vi "GPSPathTracker.vi"() -> ()   [LabVIEW 2024]
uses:
  <vilib>/Instr/_visa.llb/VISA Configure Serial Port (Instr).vi
  <vilib>/Utility/file.llb/Read Delimited Spreadsheet (DBL).vi
panel:
  in  "Steer Selector":enum32{"Stanley Method", "Pure Pursuit"}(radio)
  in  "Ld(m)":dbl=2.5 format="%#_13g"
  out "GPS":T1(graph)
  out "Tracking_Err(m)":dbl
  out "GPS_Steer_CMD(Deg)":dbl
  in  "Input_Spd(kph)":dbl
  out "RDDF_Velocity":dbl
  out "Output_Spd_CMD(%)":dbl
  out "Path_lat_arr":dbl[](array[numeric])
  out "Path_long_arr":dbl[](array[numeric])
  out "Path_Vel_arr":dbl[](array[numeric])
  out "WP_no.":i32
  out "Path_Evt_arr":dbl[](array[numeric])
  out "Evt":dbl
  in  "Map Refresh":bool
  out "X_lat_path_Full":dbl[](array[numeric])
  out "vel. path":dbl[](array[numeric])
  out "Y_long_path_Full":dbl[](array[numeric])
  out "Evt.Arr":dbl[](array[numeric])
  in  "COM7":refnum<visa-resource-name>="COM3" caption="GPS_Com."
  out "GPS_Speed(kph)":dbl format="%#_g kph"
  out "UTM Y(N) INS":dbl format="%#_13g"
  out "UTM X(E) INS":dbl format="%#_13g"
  out "True_Heading(deg)":dbl format="%#_15g"
  out "Latitude(deg)":dbl
  out "Logitude(deg)":dbl
  out "Altitude(m)":dbl
  in  "Stop":bool
  in  "RDDF":path=path "C:/Users/JungiHong/OneDrive/Hongik/HI-RACE/2026-01/ExperimentModules/GPSPathTracking/230305.txt"
  in  "k(Gain)":dbl=1.0 format="%#_13g"
  out "yi1":dbl=4158092.273483
  out "xi1":dbl=316694.021153
  out "yi":dbl=4158092.273483
  out "xi":dbl=316694.021153
  out "NMEA_Raw_Data":string
  out "CTE":dbl=20.227725199184242
  # "GPS 연결 포트"
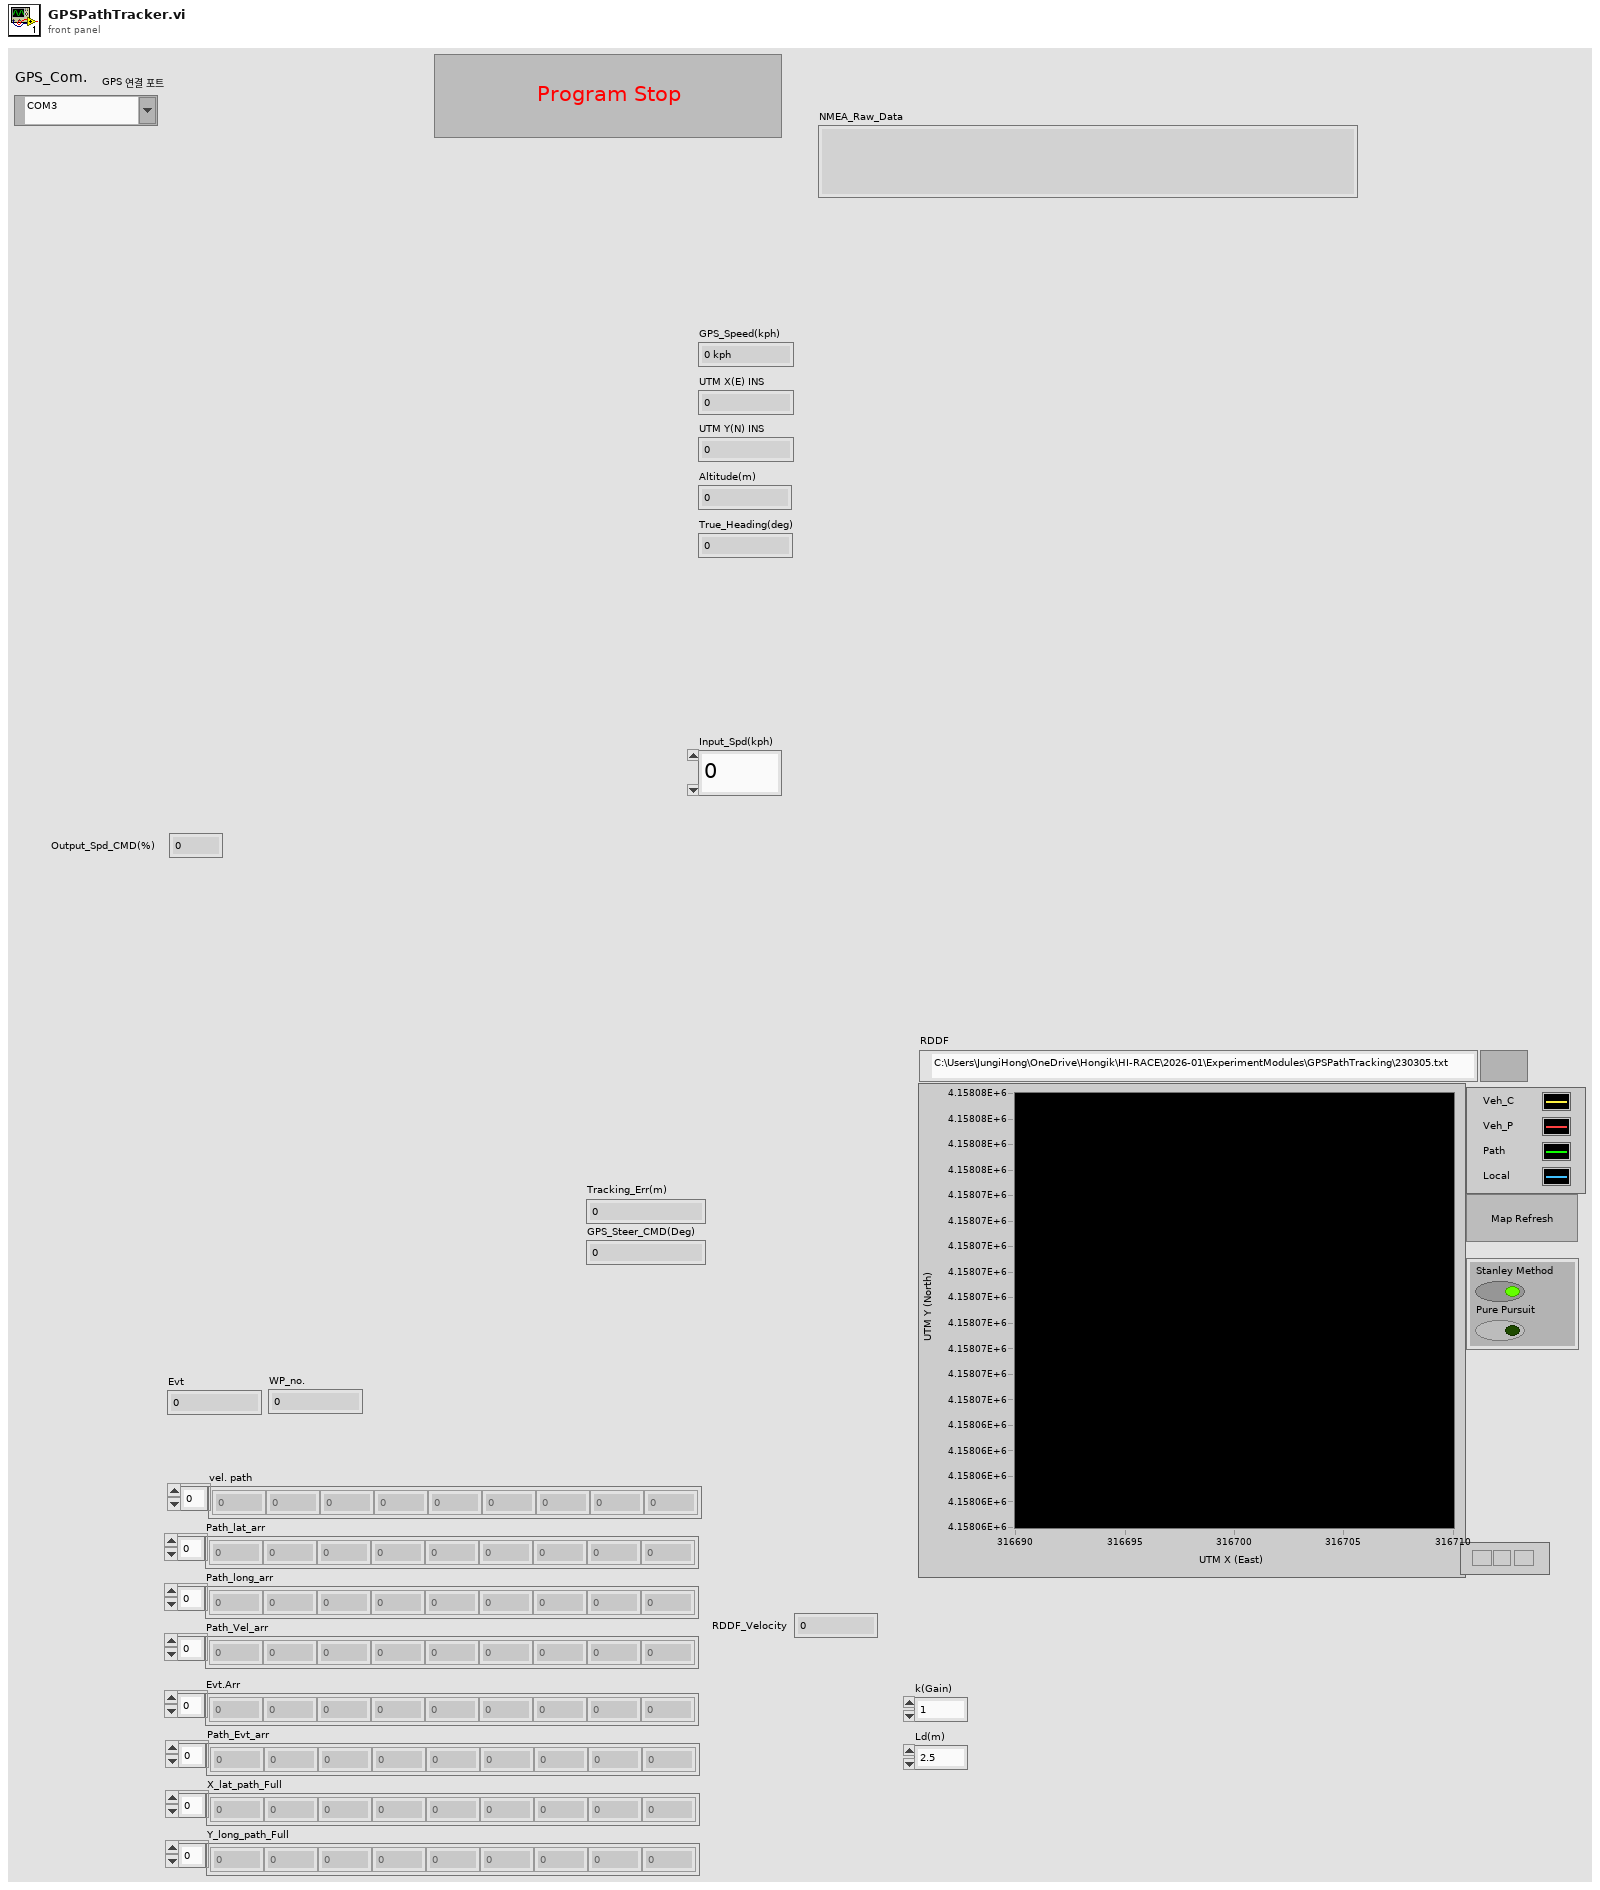
[diagram p1: front panel]
types:
  T1 = cluster{"y_long_path":dbl[], "x_lat_path":dbl[]}[]
  T2 = cluster{"oldest read timestamp":dbl, "latitude (deg)":dbl, "longitude (deg)":dbl, "ground speed (kph)":dbl, "true track angle (deg)":dbl, "altitude above mean sea level (m)":dbl}
  T3 = cluster{"X_lat_path_Full":dbl[], "Y_long_path_Full":dbl[]}
  T4 = cluster{"Path_lat_arr":dbl[], "Path_long_arr":dbl[]}
  T5 = cluster{"Path_lat_arr":dbl[], "Path_long_arr":dbl[]}[]
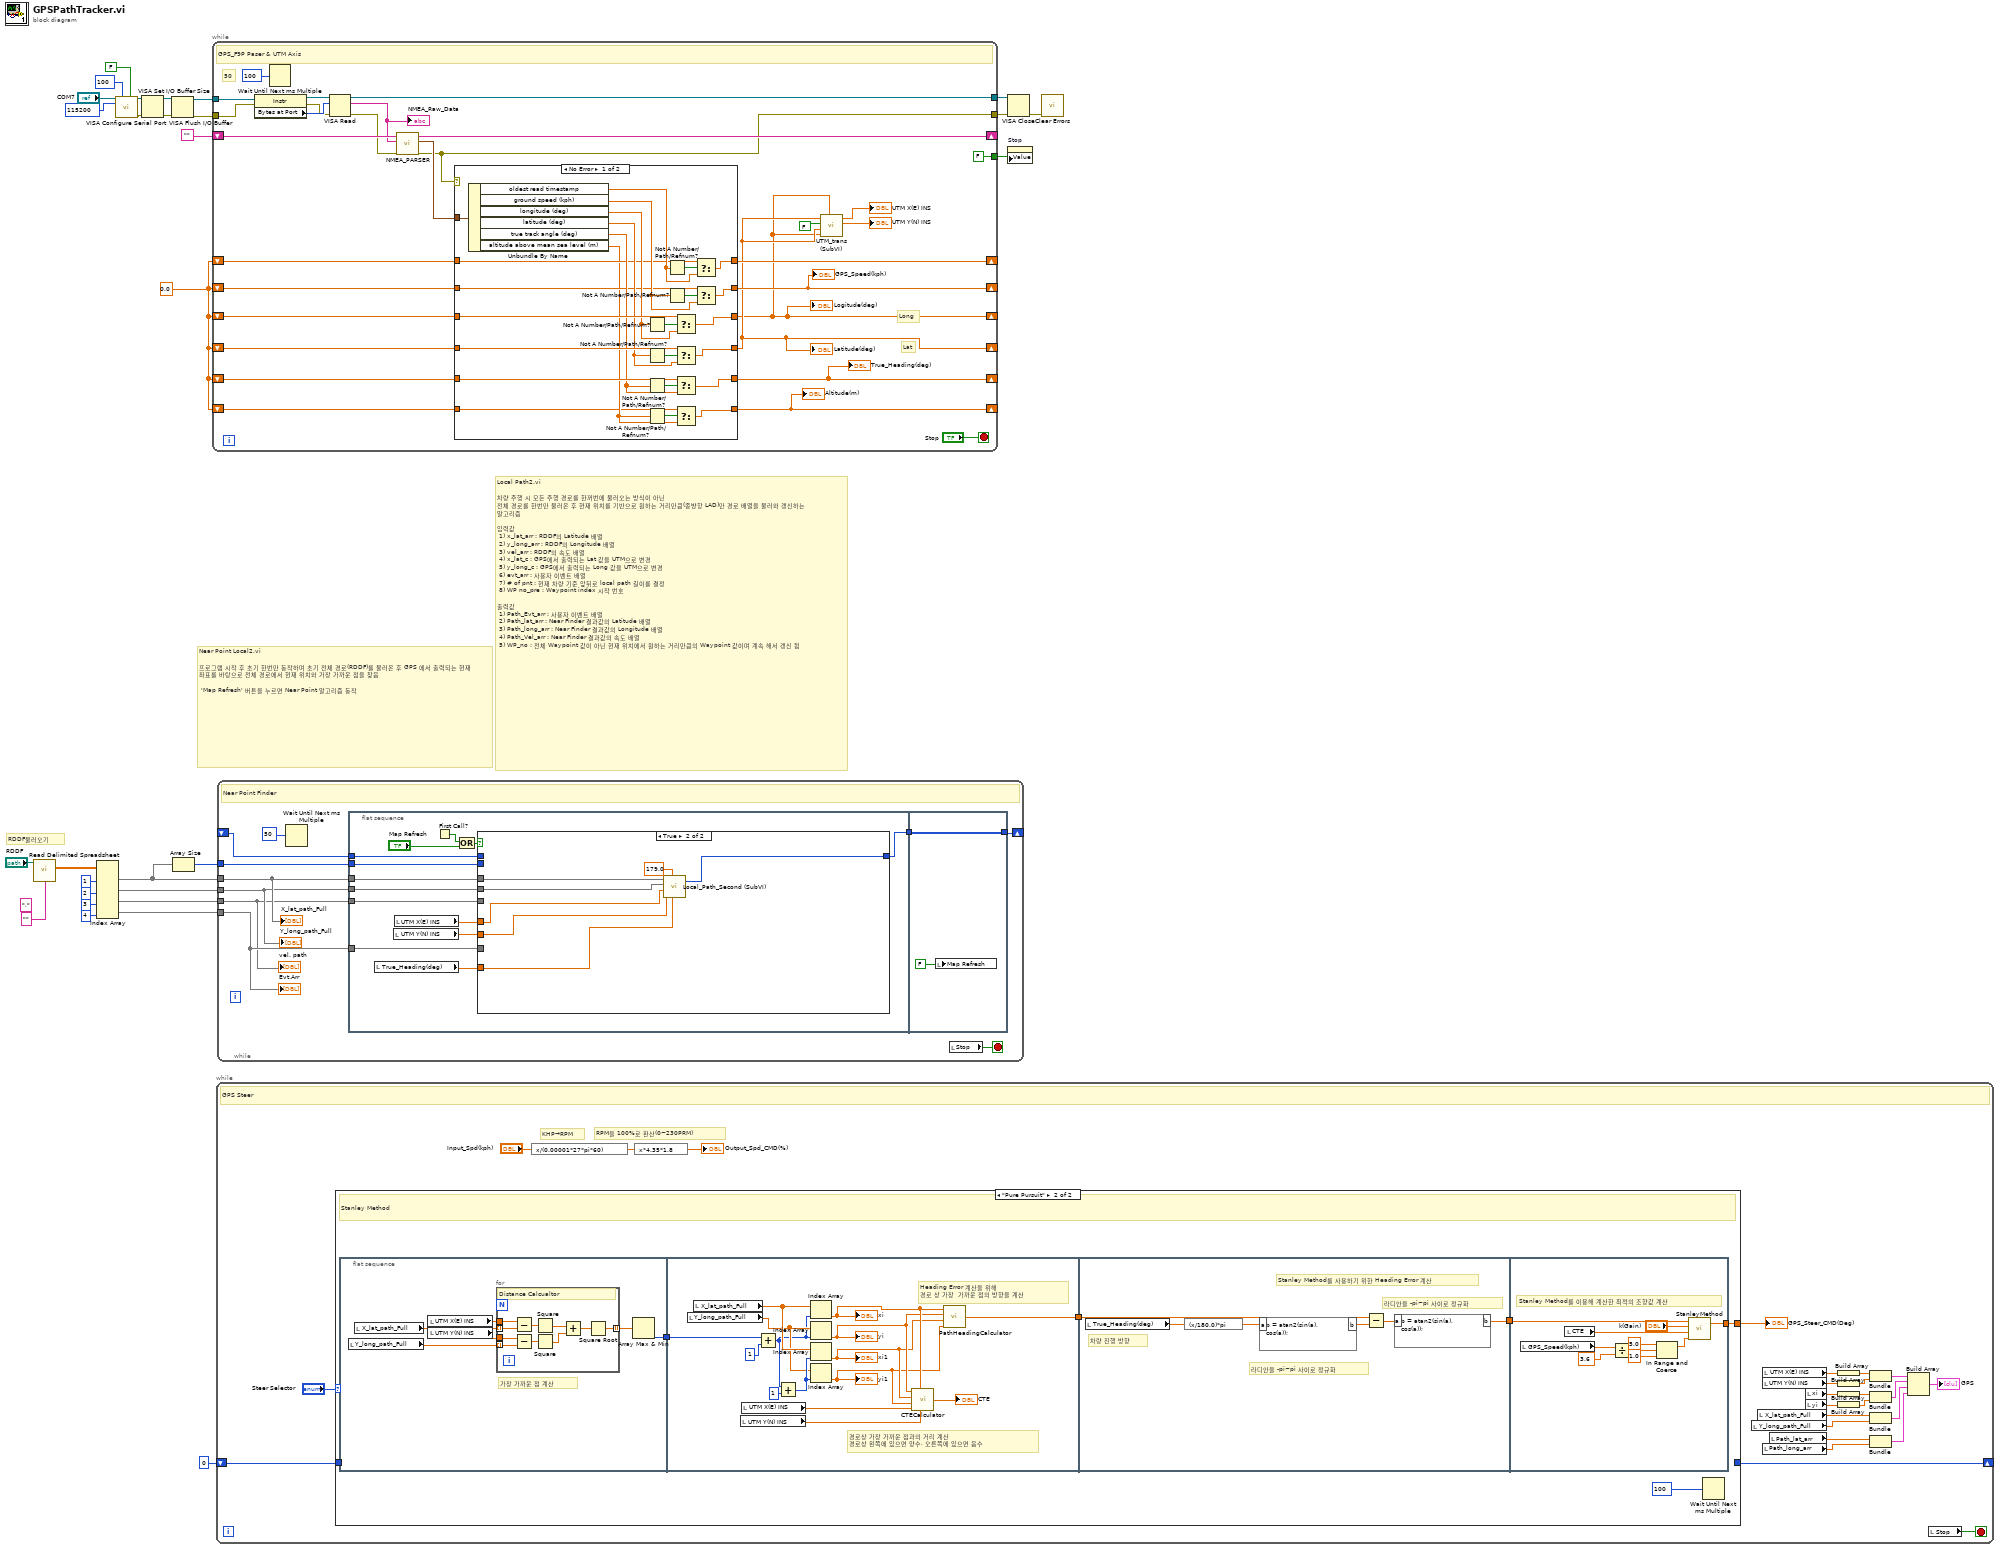
[diagram p0: block diagram]
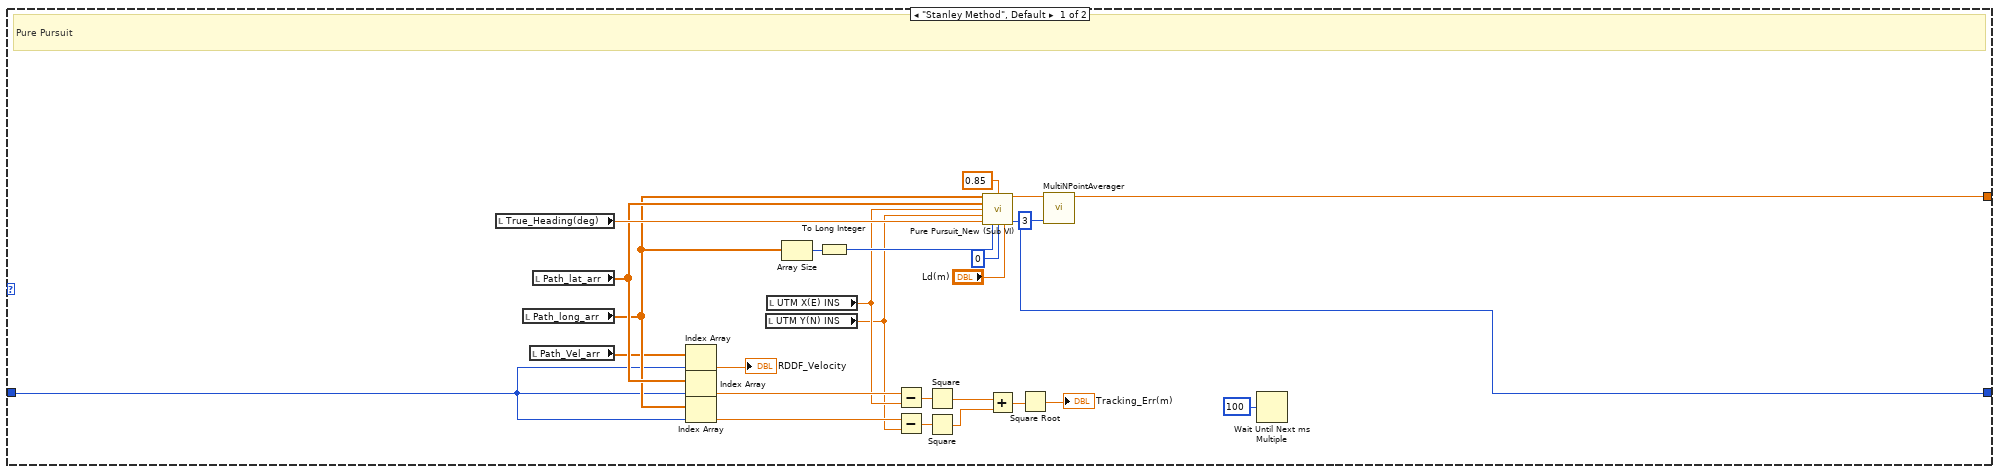
[diagram p2: hidden frame]
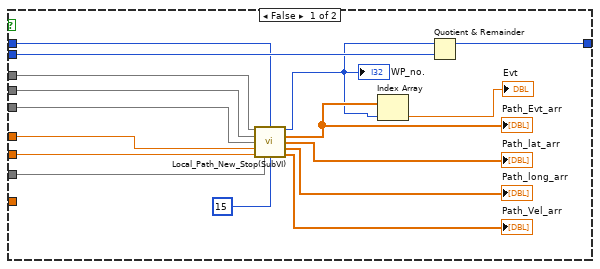
[diagram p3: hidden frame]
diagram:
  (unwired) "," ("delimiter (\\t)")
  w14 = 0.0 ("x")
  # "Near Point Local2.vi\n\n프로그램 시작 후 초기 한번만 동작하며 초기 전체 경로(RDDF)를 불러온 후 GPS 에서 출력되는 현재 좌표를 바탕으로 전체 경로에서 현재 위치와 가장 가까운 점을 찾음\n\n 'Map Refresh' 버튼을 누르면 Near Point 알고리즘 동작"
  # "Local Path2.vi\n\n차량 주행 시 모든 주행 경로를 한꺼번에 불러오는 방식이 아닌\n전체 경로를 한번만 불러온 후 현재 위치를 기반으로 원하는 거리만큼(종뱡항 LAD)만 경로 배열을 불러와 갱신하는 알고리즘\n\n입력값 \n 1) x_lat_arr : RDDF의 Latitude 배열\n 2) y_long_arr : RDDF의 Longitude 배열\n 3) vel_arr : RDDF의 속도 배열\n 4) x_lat_c : GPS에서 출력되는 Lat 값을 UTM으로 변경\n 5) y_long_c : GPS에서 출력되는 Long 값을 UTM으로 변경\n 6) evt_arr : 사용자 이벤트 배열\n 7) # of pnt : 현재 차량 기준 앞뒤로 local path 길이를 결정\n 8) WP no_pre : Waypoint index 시작 번호\n\n출력값 \n 1) Path_Evt_arr : 사용자 이벤트 배열\n 2) Path_lat_arr : Near Finder 결과값의 Latitude 배열\n 3) Path_long_arr : Near Finder 결과값의 Longitude 배열\n 4) Path_Vel_arr : Near Finder 결과값의 속도 배열\n 5) WP_no : 전체 Waypoint 값이 아닌 현재 위치에서 원하는 거리만큼의 Waypoint 값이며 계속 해서 갱신 됨"
  # "RDDF불러오기"
  n1 = call-poly <vilib>:"Read Delimited Spreadsheet.vi"("file path (dialog if empty)"="RDDF", "delimiter (\\t)"="" ("delimiter (\\t)")) -> ("all rows"=w8:dbl[][])  [unwired: 8 in, 5 out]
  n2 = Index Array(array=w8, index (col) #1=1 ("비활성화된 인덱스 (열)"), index (col) #2=2 ("인덱스 (열)"), index (col) #3=3 ("인덱스 (열)"), index (col) #4=4 ("인덱스 (열)")) -> (element #1=w5:dbl[], element #2=w4:dbl[], element #3=w2:dbl[], element #4=w3:dbl[])  [unwired: 4 in]
  n3 = call-poly "VISA Configure Serial Port"("VISA resource name"="COM7", "timeout (10sec)"=u32 100, "Enable Termination\nChar (T)"=FALSE ("Enable Termination\nChar (T)"), "baud rate (9600)"=u32 115200) -> ("VISA resource name out"=w20:refnum<visa-resource-name>, "error out"=w19:errorcluster)  [unwired: 10 in]
  n4 = VISA Set I/O Buffer Size(VISA resource name=w20, error in (no error)=w19) -> (VISA resource name out=w26:refnum<visa-resource-name>, error out=w25:errorcluster)  [unwired: 2 in]
  n5 = VISA Flush I/O Buffer(VISA resource name=w26, error in (no error)=w25) -> (VISA resource name out=w24:refnum<visa-resource-name>, error out=w23:errorcluster)  [unwired: 1 in]
  n6 = Array Size(array=w5) -> (size(s)=w6:i32)
  n7 = while {
    tunnel: w24 -> [w57]
    tunnel: w23 -> [w55]
    tunnel: [w59] -> w29
    tunnel: [w47] -> w27
    shift-right: [w48] -> _
    shift-left: "" -> [w52]
    shift-right: [w34] -> _
    shift-left: w14 -> [w46]
    shift-right: [w32] -> _
    shift-left: w14 -> [w45]
    shift-right: [w33] -> _
    shift-left: w14 -> [w44]
    shift-right: [w40] -> _
    shift-left: w14 -> [w43]
    shift-right: [w39] -> _
    shift-left: w14 -> [w42]
    tunnel: [FALSE] -> w21
    shift-right: [w30] -> _
    shift-left: w14 -> [w31]
    stop <- "Stop" stop-if-true
    # "Lat"
    # "Long"
    # "50"
    # "GPS_F9P Paser & UTM Axis"
    n8 = property class="Instr"(reference=w57, error in=w55) -> (reference out=w56:refnum<visa-resource-name>, error out=w54:errorcluster, "Bytes at Port"=w58:u32)
    n9 = Wait Until Next ms Multiple(millisecond multiple=u32 100) -> ()  [unwired: 1 out]
    n10 = VISA Read(VISA resource name=w56, byte count=w58, error in (no error)=w54) -> (VISA resource name out=w59:refnum<visa-resource-name>, read buffer=w51:string, error out=w49:errorcluster)  [unwired: 1 out]
    "NMEA_Raw_Data" <- w51
    n11 = call "NMEA_PARSER.vi"("previous partial sentence"=w52, "sensor data"=w51, "error in (no error)"=w49) -> ("remaining partial sentence"=w48:string, "GPS data"=w50:T2, "error out"=w47:errorcluster)  [unwired: 5 in]
    n12 = case shown="No Error" w47 {
      tunnel: w50 -> [w84 _]
      tunnel: w45 -> [w80 w90]
      tunnel: w44 -> [w79 w89]
      tunnel: w43 -> [w78 w88]
      tunnel: [w74 w90] -> w32
      tunnel: [w73 w89] -> w33
      tunnel: [w72 w88] -> w40
      tunnel: w46 -> [w69 w87]
      tunnel: [w68 w87] -> w34
      tunnel: w42 -> [w65 w86]
      tunnel: [w64 w86] -> w39
      tunnel: [w61 w85] -> w30
      tunnel: w31 -> [w60 w85]
      frame No Error {
        n13 = Unbundle By Name(w84) -> ("oldest read timestamp"=w66:dbl, "ground speed (kph)"=w70:dbl, "longitude (deg)"=w77:dbl, "latitude (deg)"=w76:dbl, "true track angle (deg)"=w75:dbl, "altitude above mean sea level (m)"=w62:dbl)
        n14 = Not A Number/Path/Refnum?(number/path/refnum=w77) -> (NaN/Path/Refnum?=w83:bool)
        n15 = Not A Number/Path/Refnum?(number/path/refnum=w76) -> (NaN/Path/Refnum?=w82:bool)
        n16 = Not A Number/Path/Refnum?(number/path/refnum=w75) -> (NaN/Path/Refnum?=w81:bool)
        n17 = Not A Number/Path/Refnum?(number/path/refnum=w62) -> (NaN/Path/Refnum?=w63:bool)
        n18 = Not A Number/Path/Refnum?(number/path/refnum=w66) -> (NaN/Path/Refnum?=w67:bool)
        n19 = Not A Number/Path/Refnum?(number/path/refnum=w70) -> (NaN/Path/Refnum?=w71:bool)
        n20 = Select(t=w80, s=w83, f=w77) -> (s? t:f=w74:dbl)
        n21 = Select(t=w79, s=w82, f=w76) -> (s? t:f=w73:dbl)
        n22 = Select(t=w78, s=w81, f=w75) -> (s? t:f=w72:dbl)
        n23 = Select(t=w60, s=w63, f=w62) -> (s? t:f=w61:dbl)
        n24 = Select(t=w65, s=w67, f=w66) -> (s? t:f=w64:dbl)
        n25 = Select(t=w69, s=w71, f=w70) -> (s? t:f=w68:dbl)
      }
      frame Error {
        # "Invalid data points."
      }
    }
    "True_Heading(deg)" <- w40
    "GPS_Speed(kph)" <- w34
    "Latitude(deg)" <- w33
    "Logitude(deg)" <- w32
    "Altitude(m)" <- w30
    n26 = call "UTM_trans (SubVI).vi"("Long_Deg"=w32, "long"=w32, "lat"=w33, "East?West?"=FALSE, "Lat_Deg"=w33) -> ("UTM_Y(Northing)"=→"UTM Y(N) INS":dbl, "UTM_X(Easting)"=→"UTM X(E) INS":dbl)  [unwired: 2 out]
  }
  n27 = while {
    shift-right: [w95] -> _
    shift-left: 0 ("Index(near vehicle)") -> [w94]
    stop <- w92 stop-if-true
    # "RPM을 100%로 환산(0~230PRM)"
    # "KHP→RPM"
    # "GPS Steer"
    n28 = case shown="\"Pure Pursuit\"" "Steer Selector" {
      tunnel: [w141 w142] -> w93
      tunnel: [w117 _] -> w95
      tunnel: w94 -> [w116 _]
      frame "Stanley Method", Default {
        # "Pure Pursuit"
        n29 = local read "True_Heading(deg)"() -> (w123:dbl)
        n30 = local read "Path_long_arr"() -> (w119:dbl[])
        n31 = local read "Path_Vel_arr"() -> (w118:dbl[])
        n32 = local read "Path_lat_arr"() -> (w120:dbl[])
        n33 = Index Array(array=w118, index=w116) -> (element=→"RDDF_Velocity":dbl)
        n34 = Index Array(array=w120, index=w116) -> (element=w140:dbl)
        n35 = Index Array(array=w119, index=w116) -> (element=w139:dbl)
        n36 = local read "UTM Y(N) INS"() -> (w121:dbl)
        n37 = local read "UTM X(E) INS"() -> (w122:dbl)
        n38 = Array Size(array=w119) -> (size(s)=w132:i32)
        n39 = To Long Integer(number=w132) -> (32bit integer=w131:i32)
        n40 = Subtract(x=w140, y=w122) -> (x-y=w138:dbl)
        n41 = Subtract(x=w139, y=w121) -> (x-y=w137:dbl)
        n42 = Square(x=w138) -> (x^2=w136:dbl)
        n43 = Square(x=w137) -> (x^2=w135:dbl)
        n44 = call "Pure Pursuit_New (Sub VI).vi"("x_lat_path"=w119, "L"=0.85, "y_long_path"=w120, "X_Current"=w122, "Y_Current"=w121, "Heading_Current"=w123, "#pnt"=w131, "WP no_pre"=0, "LAD"="Ld(m)") -> ("Steer_CMD(Deg)"=w127:dbl, "Index(near vehicle)"=w117:i32)  [unwired: 3 in, 2 out]
        n45 = Add(x=w136, y=w135) -> (x+y=w134:dbl)
        n46 = Square Root(x=w134) -> (sqrt(x)=→"Tracking_Err(m)":dbl)
        n47 = call "MultiNPointAverager.vi"("N point average"=3 ("WP no_pre"), "Data_input"=w127) -> ("숫자형"=w141:dbl)  [unwired: 9 in]
        n48 = Wait Until Next ms Multiple(millisecond multiple=u32 100 ("ms 배수")) -> ()  [unwired: 1 out]
      }
      frame "Pure Pursuit" {
        # "Stanley Method"
        n49 = flat-sequence {
          tunnel: [w147] -> w145
          tunnel: w145 -> [w164]
          tunnel: [w163] -> w144
          tunnel: w144 -> [w179]
          tunnel: [w178] -> w143
          tunnel: w143 -> [w185]
          tunnel: [w184] -> w142
          frame #0 {
            # "가장 가까운 점 계산"
            n50 = local read "Y_long_path_Full"() -> (w151:dbl[])
            n51 = local read "X_lat_path_Full"() -> (w150:dbl[])
            n52 = local read "UTM X(E) INS"() -> (w148:dbl)
            n53 = local read "UTM Y(N) INS"() -> (w149:dbl)
            n54 = for {
              tunnel: w148 -> [w162]
              tunnel: w149 -> [w161]
              tunnel: w150 -> [w153] mode=indexing
              tunnel: w151 -> [w154] mode=indexing
              tunnel: [w155] -> w152 mode=indexing
              # "Distance Calcualtor"
              n55 = Subtract(x=w162, y=w153) -> (x-y=w160:dbl)
              n56 = Subtract(x=w161, y=w154) -> (x-y=w159:dbl)
              n57 = Square(x=w160) -> (x^2=w158:dbl)
              n58 = Square(x=w159) -> (x^2=w157:dbl)
              n59 = Add(x=w158, y=w157) -> (x+y=w156:dbl)
              n60 = Square Root(x=w156) -> (sqrt(x)=w155:dbl)
            }
            n61 = Array Max & Min(array=w152) -> (min index (indices)=w147:i32)  [unwired: 3 out]
          }
          frame #1 {
            # "경로상 가장 가까운 점과의 거리 계산\n경로상 왼쪽에 있으면 양수, 오른쪽에 있으면 음수"
            # "Heading Error 계산을 위해\n경로 상 가장  가까운 점의 방향을 계산"
            n62 = local read "Y_long_path_Full"() -> (w172:dbl[])
            n63 = local read "X_lat_path_Full"() -> (w173:dbl[])
            n64 = local read "UTM Y(N) INS"() -> (w176:dbl)
            n65 = local read "UTM X(E) INS"() -> (w177:dbl)
            n66 = Add(x=w164, y=1) -> (x+y=w171:i32)
            n67 = Add(x=w171, y=1) -> (x+y=w175:i32)
            n68 = Index Array(array=w173, index=w171) -> (element=w170:dbl)
            "xi" <- w170
            n69 = Index Array(array=w172, index=w171) -> (element=w169:dbl)
            "yi" <- w169
            n70 = Index Array(array=w173, index=w175) -> (element=w168:dbl)
            "xi1" <- w168
            n71 = Index Array(array=w172, index=w175) -> (element=w167:dbl)
            "yi1" <- w167
            n72 = call "CTECalculator.vi"("yp"=w176, "xi"=w170, "xp"=w177, "yi1"=w167, "xi1"=w168, "yi"=w169) -> ("CTE"=→"CTE":dbl)
            n73 = call "PathHeadingCalculator.vi"("yi1"=w167, "xi1"=w168, "yi"=w169, "xi"=w170) -> ("PathHeading"=w163:dbl)
          }
          frame #2 {
            # "차량 진행 방향"
            # "Stanley Method를 사용하기 위한 Heading Error 계산"
            # "라디안을 -pi~pi 사이로 정규화"
            # "라디안을 -pi~pi 사이로 정규화"
            n74 = local read "True_Heading(deg)"() -> (w180:dbl)
            n75 = expression code="(x/180.0)*pi" ("degrees to radians")(w180) -> (w182:dbl)
            n76 = formula code="b = atan2(sin(a), cos(a));"("a"=w182) -> ("b"=w181:dbl)
            n77 = Subtract(x=w179, y=w181) -> (x-y=w183:dbl)
            n78 = formula code="b = atan2(sin(a), cos(a));"("a"=w183) -> ("b"=w178:dbl)
          }
          frame #3 {
            # "Stanley Method를 이용해 계산한 최적의 조향값 계산"
            n79 = local read "GPS_Speed(kph)"() -> (w193:dbl)
            n80 = local read "CTE"() -> (w189:dbl)
            n81 = Divide(x=w193, y=3.6) -> (x/y=w192:dbl)
            n82 = In Range and Coerce(upper limit=5.0, x=w192, lower limit=1.0) -> (coerced(x)=w191:dbl)  [unwired: 1 out]
            n83 = call "StanleyMethod.vi"("v(Velocity)m/s"=w191, "e(Cross-Track Err)m/s"=w189, "k(Gain)"="k(Gain)", "ψ(Heading Err)radian"=w185) -> ("δ(OutputSteer)degrees"=w184:dbl)  [unwired: 1 out]
          }
        }
        n84 = Wait Until Next ms Multiple(millisecond multiple=u32 100) -> ()  [unwired: 1 out]
      }
    }
    "GPS_Steer_CMD(Deg)" <- w93
    n85 = expression code="x/(0.00001*27*pi*60)"("Input_Spd(kph)") -> (w114:dbl)
    n86 = expression code="x*4.35*1.8"(w114) -> (→"Output_Spd_CMD(%)":dbl)
    n87 = local read "Y_long_path_Full"() -> (w111:dbl[])
    n88 = local read "X_lat_path_Full"() -> (w112:dbl[])
    n89 = local read "UTM Y(N) INS"() -> (w109:dbl)
    n90 = local read "Path_long_arr"() -> (w105:dbl[])
    n91 = local read "UTM X(E) INS"() -> (w110:dbl)
    n92 = local read "Path_lat_arr"() -> (w106:dbl[])
    n93 = local read "xi"() -> (w104:dbl)
    n94 = local read "yi"() -> (w103:dbl)
    n95 = Build Array(w110) -> (w108:dbl[])
    n96 = Build Array(w109) -> (w107:dbl[])
    n97 = Build Array(w104) -> (w102:dbl[])
    n98 = Build Array(w103) -> (w101:dbl[])
    n99 = Bundle(w108, w107) -> (w100:cluster{dbl[], dbl[]})  [unwired: 1 in]
    n100 = Bundle(w102, w101) -> (w99:cluster{dbl[], dbl[]})  [unwired: 1 in]
    n101 = Bundle("X_lat_path_Full"=w112, "Y_long_path_Full"=w111) -> (w98:T3)  [unwired: 1 in]
    n102 = Bundle("Path_lat_arr"=w106, "Path_long_arr"=w105) -> (w97:T4)  [unwired: 1 in]
    n103 = Build Array(w100, w99, w98, w97) -> (→"GPS":T5)
    n104 = local read "Stop"() -> (w92:bool)
  }
  n105 = while {
    shift-right: [w202] -> _
    shift-left: _ -> [w203]
    tunnel: w6 -> [w200]
    tunnel: w2 -> [w194]
    tunnel: w4 -> [w195]
    tunnel: w5 -> [w196]
    tunnel: w3 -> [w199]
    stop <- w198 stop-if-true
    # "Near Point Finder"
    n106 = Wait Until Next ms Multiple(millisecond multiple=u32 50) -> ()  [unwired: 1 out]
    n107 = flat-sequence {
      tunnel: [w215] -> w201
      tunnel: w203 -> [w216]
      tunnel: w200 -> [w211]
      tunnel: w194 -> [w210]
      tunnel: w195 -> [w209]
      tunnel: w196 -> [w208]
      tunnel: w199 -> [w207]
      tunnel: [w241] -> w202
      tunnel: w201 -> [w241]
      frame #0 {
        n108 = local read "True_Heading(deg)"() -> (w204:dbl)
        n109 = local read "UTM Y(N) INS"() -> (w205:dbl)
        n110 = local read "UTM X(E) INS"() -> (w206:dbl)
        n111 = First Call?() -> (First Call?: T/F=w213:bool)
        n112 = Or(x=w213, y="Map Refresh") -> (x .or. y?=w214:bool)
        n113 = case shown="True" w214 {
          tunnel: w208 -> [w228 w239]
          tunnel: w209 -> [w229 w238]
          tunnel: w216 -> [w227 _]
          tunnel: w210 -> [w230 _]
          tunnel: w211 -> [w231 _]
          tunnel: [w232 w236] -> w215
          tunnel: w207 -> [w222 _]
          tunnel: w206 -> [w221 w235]
          tunnel: w205 -> [w220 w234]
          tunnel: w204 -> [_ w233]
          frame False {
            n114 = call "Local_Path_New_Stop(SubVI).vi"("x_lat_arr"=w228, "WP no_pre"=w227, "y_long_arr"=w229, "vel_arr"=w230, "x_lat_c"=w221, "y_long_c"=w220, "evt_arr"=w222, "# of pnt"=15) -> ("INDEX(Near Point)"=w218:i32, "Evt(Local)"=w224:dbl[], "Lat(Local)"=→"Path_lat_arr":dbl[], "Long(Local)"=→"Path_long_arr":dbl[], "Vel(Local)"=→"Path_Vel_arr":dbl[])  [unwired: 3 in]
            "WP_no." <- w218
            "Path_Evt_arr" <- w224
            n115 = Index Array(array=w224, index=w218) -> (element=→"Evt":dbl)
            n116 = Quotient & Remainder(x=w218, y=w231) -> (x-y*floor(x/y)=w232:i32)  [unwired: 1 out]
          }
          frame True {
            n117 = call "Local_Path_Second (SubVI).vi"("heading_deg"=w233, "heading_limit"=179.0, "y_long"=w234, "x_lat"=w235, "Y_long_path"=w238, "X_lat_path"=w239) -> ("Index(near vehicle)"=w236:i32)  [unwired: 1 out]
          }
        }
      }
      frame #1 {
        n118 = local write "Map Refresh"(FALSE ("Refresh")) -> ()
      }
    }
    n119 = local read "Stop"() -> (w198:bool)
    "X_lat_path_Full" <- w196
    "vel. path" <- w194
    "Y_long_path_Full" <- w195
    "Evt.Arr" <- w199
  }
  n120 = VISA Close(VISA resource name=w29, error in (no error)=w27) -> (error out=w28:errorcluster)
  n121 = property on="Stop" class="Bool (strict)"("Value"=w21) -> ()  [unwired: 2 in, 2 out]
  n122 = call <vilib>:"Clear Errors.vi"("error in (no error)"=w28) -> ()  [unwired: 5 in, 2 out]
